vi "Raw2Angle.vi"(2 "Calibration":cluster{"Offset":dbl, "Gain":dbl}[](array[cluster]), 3 "Raw Data":u8[](array[numeric])) -> (0 "Degrees":dbl[](array[numeric]), 1 "Radians":dbl[](array[numeric]))   [LabVIEW 2012]
doc: "Takes the raw data from the cyberglove and applies the gains and offsets from the calibration array to produce the angles of all the joints in both radians and degrees"
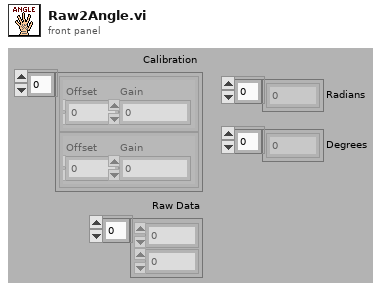
[diagram p1: front panel]
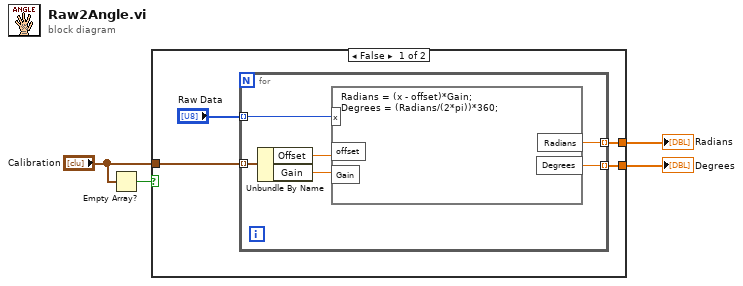
[diagram p0: block diagram]
diagram:
  n1 = Empty Array?(array="Calibration") -> (empty?=w1:bool)
  n2 = case shown="False" w1 {
    tunnel: [w7 _] -> w4
    tunnel: [w6 _] -> w3
    tunnel: "Calibration" -> [w5 _]
    frame False {
      n3 = for {
        tunnel: w5 -> [w14] mode=indexing
        tunnel: "Raw Data" -> [w11] mode=indexing
        tunnel: [w10] -> w7 mode=indexing
        tunnel: [w9] -> w6 mode=indexing
        n4 = Unbundle By Name(w14) -> ("Offset"=w13:dbl, "Gain"=w12:dbl)
        n5 = formula code="Radians = (x - offset)*Gain;\nDegrees = (Radians/(2*pi))*360;"("offset"=w13, "Gain"=w12, "x"=w11) -> ("Radians"=w10:dbl, "Degrees"=w9:dbl)
      }
    }
    frame True {
      # "If no calibration exists return empty arrays"
    }
  }
  "Radians" <- w4
  "Degrees" <- w3
